vi "GetAllDependencyClasses.vi"(8 "error in (no error)":errorcluster, 11 "SubVI in":refnum<vi>) -> (0 "error out":errorcluster, 2 "VI Name":string, 3 "Implementations JSON string":string)   [LabVIEW 2017]
uses:
  JsonConverters/GObjectConverters/SubVIConverter/DynamicDispatchJsonConstants.vi
  JsonConverters/GObjectConverters/SubVIConverter/SubVIConverter.lvclass
  JsonConverters/JsonFormatter/JsonFormatter.lvlib
  JsonConverters/TreeSerializer/TreeSerializer.lvlib
  JsonConverters/GObjectConverters/SubVIConverter/DynamicDispatch/DynamicDispatchImplementationWalker.lvlib
panel:
  in  "Class Hierarchy":string[](tree) caption="Select VI"
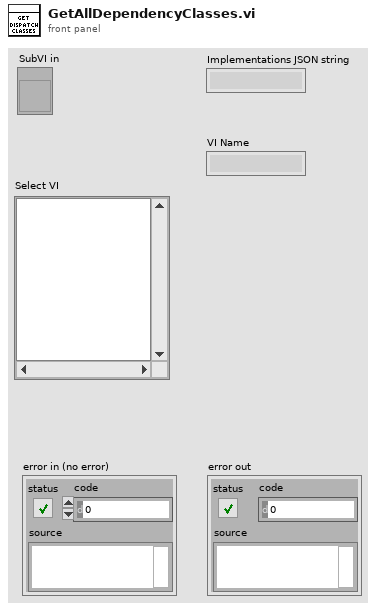
[diagram p1: front panel]
types:
  T1 = typedef "TreeSerializer.lvlib/KeyValuePair.ctl" = cluster{"Tag":string, "Path":string}
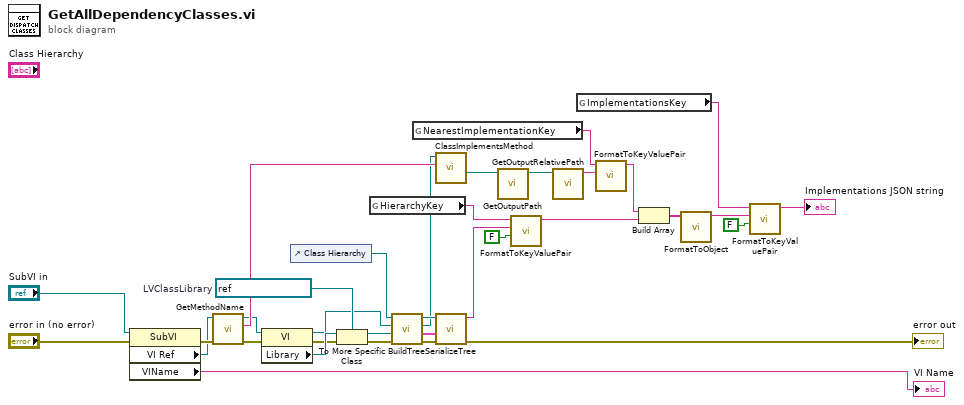
[diagram p0: block diagram]
diagram:
  w19 = refnum<vi> refnum  # LVClassLibrary
  n1 = property class="SubVI"(reference="SubVI in", error in="error in (no error)") -> (error out=w7:errorcluster, "VI Ref"=w5:refnum<vi>, "VIName"=→"VI Name":string)  [unwired: 1 out]
  n2 = call "GetMethodName.vi"("error in (no error)"=w7, "VI Reference"=w5) -> ("error out"=w6:errorcluster, "Method Name"=w11:string, "VI Reference out"=w4:refnum<vi>)  [unwired: 7 in]
  n3 = property class="VI"(reference=w4, error in=w6) -> (reference out=w12:refnum<vi>, error out=w18:errorcluster, "Library"=w20:refnum<vi>)
  n4 = control-ref of="Class Hierarchy"() -> (w22:refnum<vi>)
  n5 = To More Specific Class(target class=w19, reference=w20, error in=w18) -> (specific class reference=w13:refnum<vi>, error out=w17:errorcluster)
  n6 = global read "DynamicDispatchJsonConstants.vi" "HierarchyKey"() -> (w28:string)
  n7 = call "BuildTree.vi"("error in (no error)"=w17, "Wired-in Class Refnum"=w13, "Method Refnum"=w12, "Tree Refnum"=w22) -> ("error out"=w14:errorcluster, "Class To VI Path Map"=w2:T1[], "Nearest Implementation"=w1:refnum<vi>, "Tree Refnum out"=w21:refnum<vi>)  [unwired: 3 in, 1 out]
  n8 = global read "DynamicDispatchJsonConstants.vi" "NearestImplementationKey"() -> (w31:string)
  n9 = call "ClassImplementsMethod.vi"("Method Name"=w11, "Class Refnum"=w1) -> ("Path"=w9:path)  [unwired: 6 in, 3 out]
  n10 = call "SerializeTree.vi"("error in (no error)"=w14, "TagToPathMap"=w2, "Tree Refnum"=w21) -> ("error out"=→"error out":errorcluster, "Formatted JSON string"=w27:string)  [unwired: 7 in]
  n11 = call "GetOutputPath.vi"("Path"=w9) -> ("Output Path"=w10:path)  [unwired: 10 in]
  n12 = call "FormatToKeyValuePair.vi"("Escape Value string?"=FALSE, "Value"=w27, "Key"=w28) -> ("Formatted string"=w25:string)  [unwired: 8 in]
  n13 = call "GetOutputRelativePath.vi"("Path"=w10) -> ("Output relative path"=w8:string)  [unwired: 9 in, 1 out]
  n14 = global read "DynamicDispatchJsonConstants.vi" "ImplementationsKey"() -> (w32:string)
  n15 = call "FormatToKeyValuePair.vi"("Value"=w8, "Key"=w31) -> ("Formatted string"=w29:string)  [unwired: 9 in]
  n16 = Build Array(w29, w25) -> (w26:string[])
  n17 = call "FormatToObject.vi"("Properties"=w26) -> ("Formatted string"=w30:string)  [unwired: 10 in]
  n18 = call "FormatToKeyValuePair.vi"("Escape Value string?"=FALSE, "Value"=w30, "Key"=w32) -> ("Formatted string"=→"Implementations JSON string":string)  [unwired: 8 in]
